vi "Build Data Log File Path.vi"(8 "error in (no error)":errorcluster, 9 "Timestamp":bool, 10 "Name":string, 11 "Log File Directory":path) -> (0 "error out":errorcluster, 3 "appended path":path)   [LabVIEW 2018, in "Embedded Data Logger System Explorer.lvlib"]
uses:
  Embedded Data Logger System Explorer.lvlib
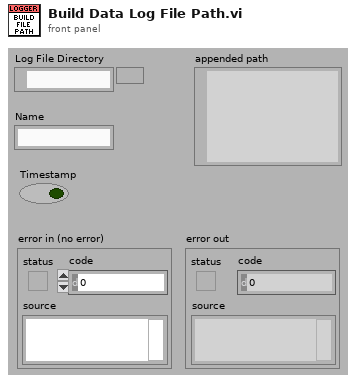
[diagram p1: front panel]
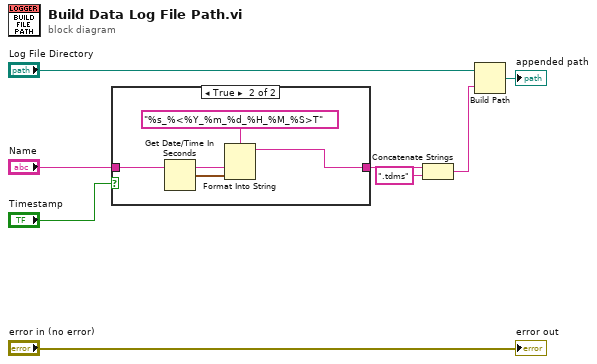
[diagram p0: block diagram]
diagram:
  n1 = case shown="True" "Timestamp" {
    tunnel: "Name" -> [w9 w13]
    tunnel: [w9 w12] -> w6
    frame False {
    }
    frame True {
      n2 = Get Date/Time In Seconds() -> (seconds since 1Jan1904=w10:timestamp)
      n3 = Format Into String(format string="%s_%<%Y_%m_%d_%H_%M_%S>T", w13, w10) -> (resulting string=w12:string)  [unwired: 2 in, 1 out]
    }
  }
  n4 = Concatenate Strings(w6, ".tdms" ("string")) -> (w8:string)
  n5 = Build Path(base path="Log File Directory", name or relative path=w8) -> (appended path=→"appended path":path)
  "error out" <- "error in (no error)"
